vi "remove_duplicates_by_column.vi"(10 "Column":i32, 11 "Array in":string[][](array[string])) -> (3 "Array out":string[][](array[string]))   [LabVIEW 2016]
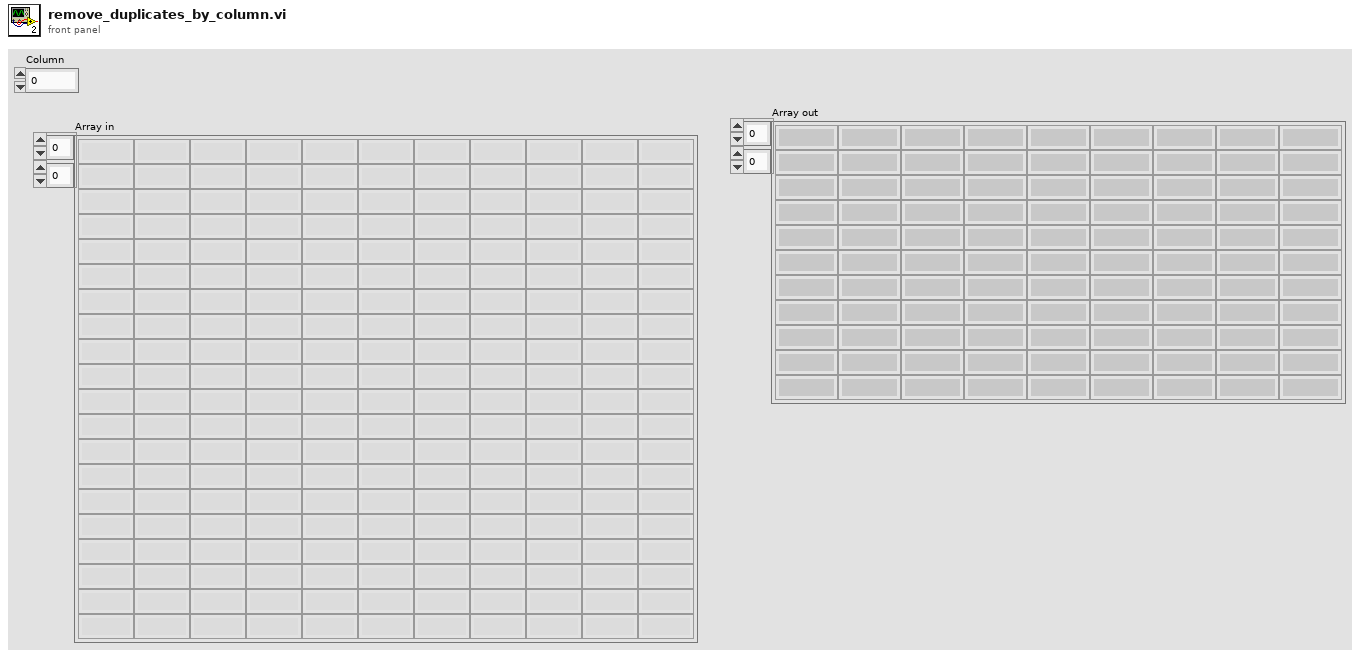
[diagram p1: front panel]
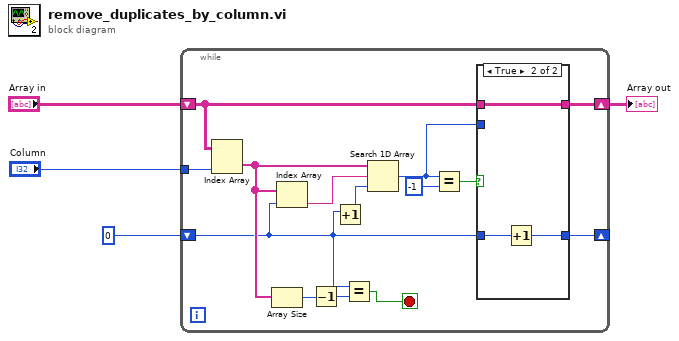
[diagram p0: block diagram]
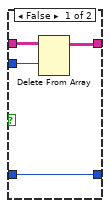
[diagram p2: hidden frame]
diagram:
  n1 = while {
    shift-right: [w14] -> w1
    shift-left: "Array in" -> [w12]
    shift-right: [w13] -> _
    shift-left: 0 ("index") -> [w6]
    tunnel: "Column" -> [w10]
    stop <- w5 stop-if-true
    n2 = Index Array(array=w12, index (col)=w10) -> (element=w11:string[])  [unwired: 1 in]
    n3 = Array Size(array=w11) -> (size(s)=w8:i32)
    n4 = Index Array(array=w11, index=w6) -> (element=w18:string)
    n5 = Decrement(x=w8) -> (x-1=w7:i32)
    n6 = Increment(x=w6) -> (x+1=w9:i32)
    n7 = Equal?(x=w6, y=w7) -> (x = y?=w5:bool)
    n8 = Search 1D Array(1D array=w11, element=w18, start index (0)=w9) -> (index of element=w15:i32)
    n9 = Equal?(x=w15, y=-1) -> (x = y?=w16:bool)
    n10 = case shown="True" w16 {
      tunnel: w12 -> [w22 w24]
      tunnel: w15 -> [w21 _]
      tunnel: w6 -> [w19 w25]
      tunnel: [w20 w24] -> w14
      tunnel: [w19 w23] -> w13
      frame False {
        n11 = Delete From Array(array=w22, index (row)=w21) -> (array with subset deleted=w20:string[][])  [unwired: 2 in, 1 out]
      }
      frame True {
        n12 = Increment(x=w25) -> (x+1=w23:i32)
      }
    }
  }
  "Array out" <- w1
